vi "UI_Device_Lubricate_Unit.vi"() -> ()   [LabVIEW 2014]
panel:
  out "DATA":T1
  in  "退出":bool
  # "陪试单元监测参数"
  # "报警信息"
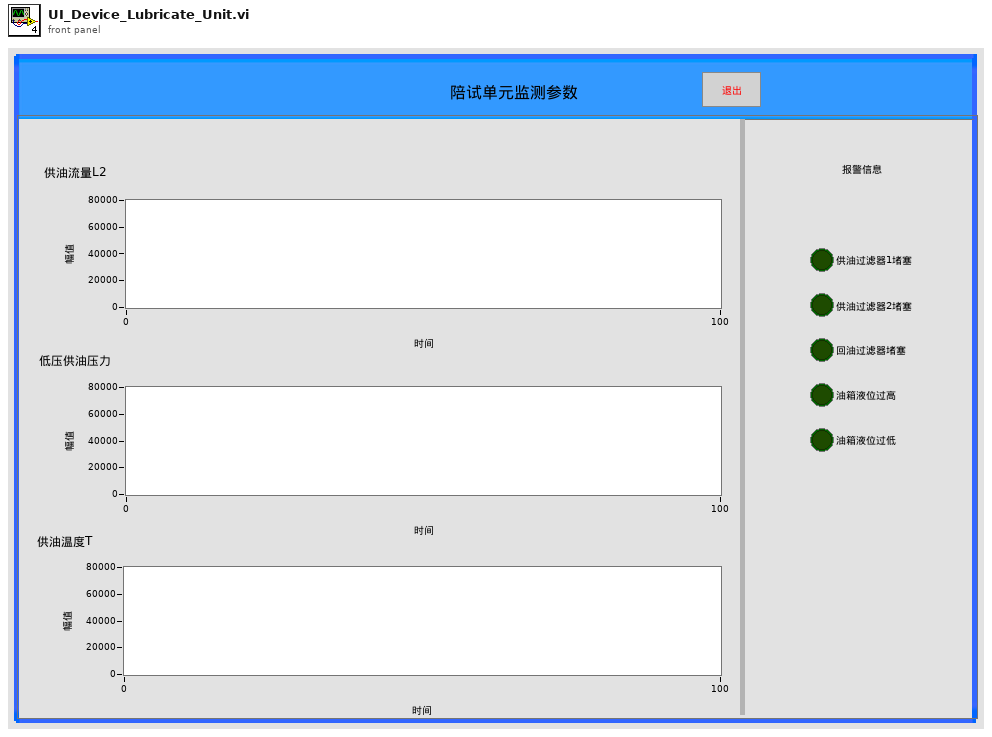
[diagram p1: front panel]
types:
  T1 = cluster{"供油流量L2":cluster{sgl, sgl, "陪试轴承供油流量":u16}, "供油压力":cluster{sgl, sgl, "陪试轴承供油压力":u16}, "供油温度T":cluster{sgl, sgl, "陪试轴承供油温度":u16}, "报警信息":cluster{"陪试轴承单元供油过滤器1堵塞":bool, "陪试轴承单元供油过滤器2堵塞":bool, "陪试轴承单元回油过滤器堵塞":bool, "陪试轴承单元油箱液位过高":bool, "陪试轴承单元油箱液位过低":bool}}
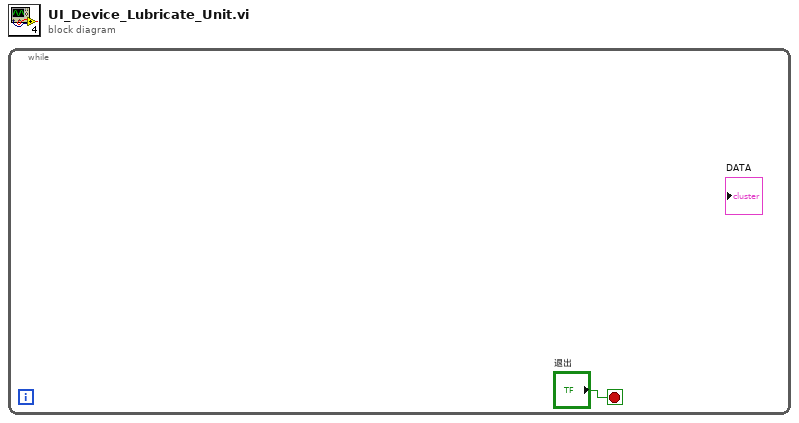
[diagram p0: block diagram]
diagram:
  n1 = while {
    stop <- "退出" stop-if-true
  }
